vi "FPGA_TimedLoopTest1.vi"() -> ()   [LabVIEW 2014]
uses:
  <vilib>/Platform/TimedLoop/XDataNode/timing_clust.ctl
  <vilib>/Platform/TimedLoop/XDataNode/nitl_modes.ctl
  <vilib>/Platform/TimedLoop/XDataNode/wakeup.ctl
  <vilib>/rvi/FXPMathLib/FxpConvert/subVIs/nifxpmath_Convert_SimConfig.ctl
  <vilib>/fxp/LVFixedPointQuantizationPolicyTypeDef.ctl
  <vilib>/fxp/LVFixedPointOverflowPolicyTypeDef.ctl
  <vilib>/rvi/Emulation/niFpgaSctlEmulationGetInTimedLoop.vi
  <vilib>/rvi/Emulation/niFpgaEmulationReportErrorSimple.vi
  <vilib>/rvi/Emulation/niFpgaGetClockAttributes.vi
  <vilib>/rvi/Emulation/niFpgaCriticalErrorInLSC.vi
  <vilib>/rvi/FXPMathLib/FxpConvert/simVIs/DllFxpConvertTemp_sub.vi
  <vilib>/Platform/TimedLoop/XDataNode/XDataNode.xnode
  <vilib>/rvi/FXPMathLib/FxpMul/XNode/nifxpmath_Multiplier.xnode
  <vilib>/rvi/FXPMathLib/FxpConvert/XNode/nifxpmath_Convert.xnode
  <vilib>/Platform/TimedLoop/XDataNode/XDNodeRunTimeDep.lvlib
  <vilib>/rvi/FXPMathLib/sim/FxpSim.dll
panel:
  out "y":fxp<+/-,16,16>
  out "TimeDelta":u32
  in  "stop":bool
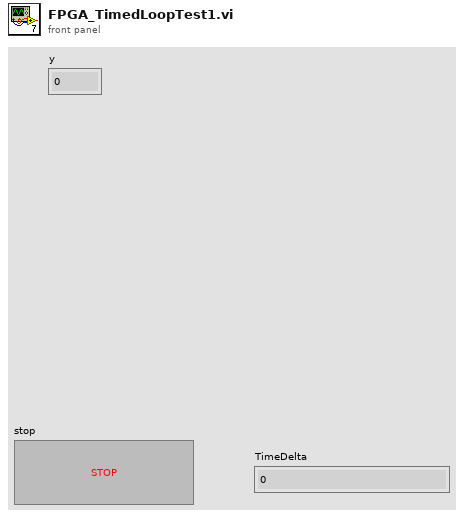
[diagram p1: front panel]
types:
  T1 = typedef "XDNodeRunTimeDep.lvlib/timing_clust.ctl" = cluster{"Expected End [f-1]":u64, "Actual End [f-1]":u64, "Finished Late? [f-1]":bool, "Expected End [i-1]":u64, "Actual End [i-1]":u64, "Finished Late? [i-1]":bool, "Expected Start [i]":u64, "Actual Start [i]":u64, "Expected Start [f]":u64, "Actual Start [f]":u64, "Source Name":string, "Structure Name":string, "Period":i64, "Deadline":i64, "Offset":i64, "Start":i64, "Priority":i32, "Timeout":i32, "Mode":T2, "Wakeup Reason":T3, "Error":errorcluster, "Source Type":string, "Secondary Source Type":string, "Global End Time":u64, "Global Start Time":u64, "Frame Duration":u64, "Iteration Duration":u64, "Assigned CPU":i32, "I/O Scan Engine Mode":u32}
  T2 = typedef "XDNodeRunTimeDep.lvlib/nitl_modes.ctl" = enum32{"No Change", "Process missed periods, maintain original phase", "Discard missed periods, maintain original phase", "Process missed periods, ignore original phase", "Discard missed periods, ignore original phase"}
  T3 = typedef "XDNodeRunTimeDep.lvlib/wakeup.ctl" = enum32{"Normal", "Aborted", "Asynchronous wakeup", "Timing source error", "Timed loop error", "Timeout"}
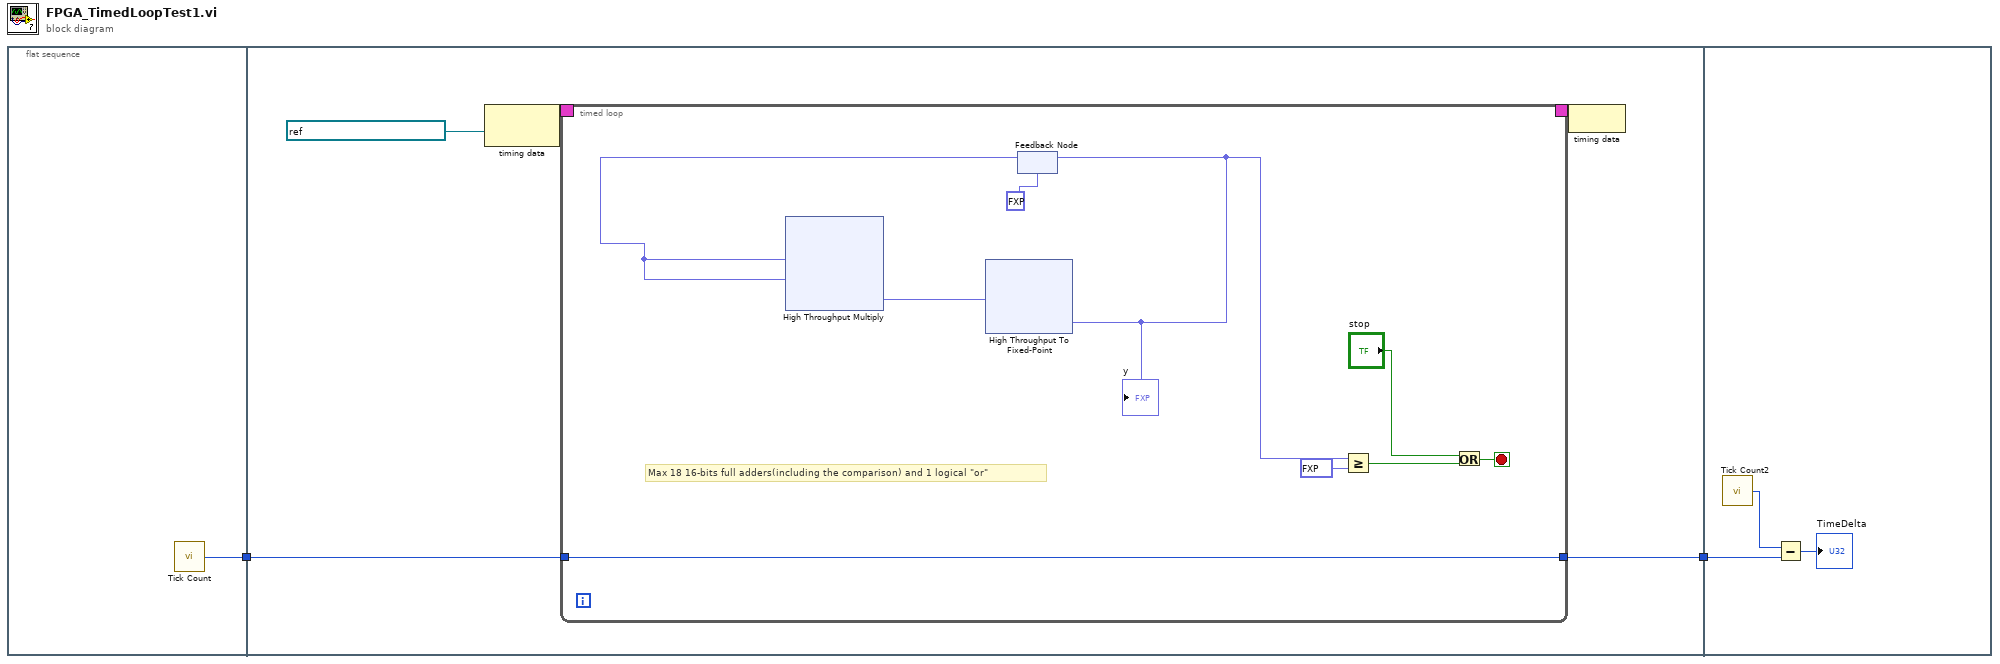
[diagram p0: block diagram]
diagram:
  n1 = flat-sequence {
    tunnel: [w3] -> w2
    tunnel: w2 -> [w5]
    tunnel: [w4] -> w1
    tunnel: w1 -> [w47]
    frame #0 {
      n2 = call "Tick Count"() -> ("Tick Count(mSec)"=w3:u32)
    }
    frame #1 {
      n3 = node-c288(refnum<k21> "40 MHz Onboard Clock" ("Source Name")) -> (w8:T1)
      n4 = timed-loop {
        timing: w8 -> [_]
        timing-out: [_] -> w7
        tunnel: w5 -> [w12]
        tunnel: [w12] -> w4
        stop <- w16 stop-if-true
        # "Max 18 16-bits full adders(including the comparison) and 1 logical \"or\""
        n5 = feedback #1(fxp<+,1,2> 2.0) -> (w11:fxp<+/-,16,10>)
        n6 = xnode ("High Throughput Multiply")("x"=w11, "y"=w11) -> ("x*y"=w10:fxp<+/-,32,20>)
        n7 = xnode ("High Throughput To Fixed-Point")("x"=w10) -> ("y"=w9:fxp<+/-,16,10>)
        "y" <- w9
        n8 = feedback-in #1(w9) -> ()
        n9 = Greater Or Equal?(x=w9, y=fxp<+,7,10> 1000.0) -> (x >= y?=w14:bool)
        n10 = Or(x="stop", y=w14) -> (x .or. y?=w16:bool)
      }
      n11 = node-c288(w7) -> ()
    }
    frame #2 {
      n12 = call "Tick Count2"() -> ("Tick Count(mSec)"=w48:u32)
      n13 = Subtract(x=w48, y=w47) -> (x-y=→"TimeDelta":u32)
    }
  }
